vi "String to Bool.vi"(3 "String":string) -> (1 "Bool":bool)   [LabVIEW 2020, in "Vecto.lvlib"]
uses:
  Vecto.lvlib
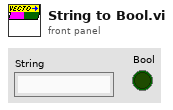
[diagram p1: front panel]
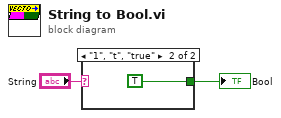
[diagram p0: block diagram]
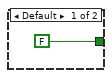
[diagram p2: hidden frame]
diagram:
  n1 = case shown="\"1\", \"t\", \"true\"" "String" {
    tunnel: [FALSE TRUE] -> w1
    frame Default {
    }
    frame "1", "t", "true" {
    }
  }
  "Bool" <- w1
